vi "Reset.vi"(8 "error in (no error)":errorcluster, 11 "VISA resource name":refnum<visa-resource-name>) -> (0 "error out":errorcluster, 3 "VISA resource name out":refnum<visa-resource-name>)   [LabVIEW 2023, in "Tti-Pl303Qmd.lvlib"]
doc: "Reset"
uses:
  Tti-Pl303Qmd.lvlib
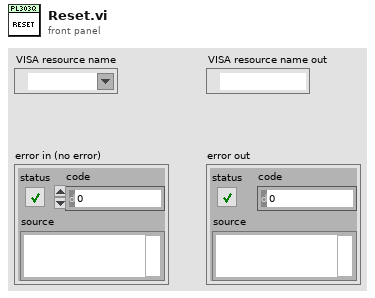
[diagram p1: front panel]
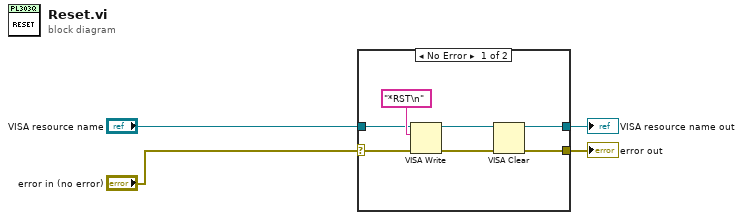
[diagram p0: block diagram]
diagram:
  n1 = case shown="No Error" "error in (no error)" {
    selector: "error in (no error)" -> [w7 w13]
    tunnel: "VISA resource name" -> [w8 w12]
    tunnel: [w9 w13] -> w4
    tunnel: [w6 w12] -> w2
    frame No Error {
      n2 = VISA Write(VISA resource name=w8, write buffer="*RST\n", error in (no error)=w7) -> (VISA resource name out=w5:refnum<visa-resource-name>, error out=w10:errorcluster)  [unwired: 1 out]
      n3 = VISA Clear(VISA resource name=w5, error in (no error)=w10) -> (VISA resource name out=w6:refnum<visa-resource-name>, error out=w9:errorcluster)
    }
    frame Error {
    }
  }
  "error out" <- w4
  "VISA resource name out" <- w2
